vi "I32.vi"(1 "Numeric Input":i32) -> (0 "Numeric Output":i32)   [LabVIEW 2011]
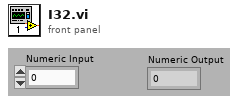
[diagram p1: front panel]
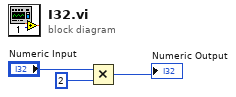
[diagram p0: block diagram]
diagram:
  n1 = Multiply(x="Numeric Input", y=2) -> (x*y=→"Numeric Output":i32)
